vi "OP300ZP_prep bdd cloture.vi"(8 "tabin":string[](array[string]), 10 "tp1904":timestamp, 11 "Ok final":bool) -> (0 "tabout":string[](array[string]))   [LabVIEW 2020]
uses:
  OP300ZP_selectdata.ctl
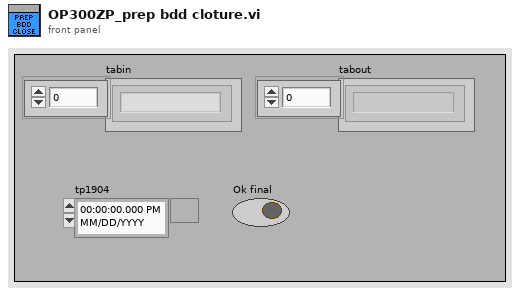
[diagram p1: front panel]
types:
  T1 = typedef "OP300ZP_selectdata.ctl" = u16
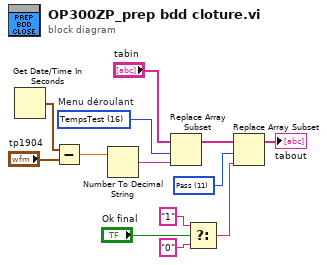
[diagram p0: block diagram]
diagram:
  w1 = T1 11 items=["IdOp300", "DateStart", "DeltaTC", "DeltaVC", "ImageVers", "IniFileVers", "InsuN", "InsuP", "MCU", "OCV", "Operateur", "Pass", "SN", "SoftVers", "TC0", "TC1", "TempsTest", "Tfactory", "Type", "VC0", "VC1"] ("Menu déroulant")
  w2 = T1 16 items=["IdOp300", "DateStart", "DeltaTC", "DeltaVC", "ImageVers", "IniFileVers", "InsuN", "InsuP", "MCU", "OCV", "Operateur", "Pass", "SN", "SoftVers", "TC0", "TC1", "TempsTest", "Tfactory", "Type", "VC0", "VC1"]  # Menu déroulant
  n1 = Get Date/Time In Seconds() -> (seconds since 1Jan1904=w7:timestamp)
  n2 = Subtract(x=w7, y="tp1904") -> (x-y=w11:dbl)
  n3 = Number To Decimal String(number=w11) -> (decimal integer string=w12:string)  [unwired: 1 in]
  n4 = Replace Array Subset(array="tabin", new element=w12, index=w2) -> (w10:string[])
  n5 = Select ("Sélectionner")(t="1", s="Ok final", f="0") -> (s? t:f=w6:string)
  n6 = Replace Array Subset(array=w10, new element=w6, index=w1) -> (→"tabout":string[])
